vi "Configure Channel Spacing.vi"(7 "error in (no error)":errorcluster {"code" format="%.0x"}, 9 "FrequencyDifference":dbl[](array[numeric])=[20000000.0, 40000000.0, 60000000.0] format="%.2p", 10 "instrument handle":refnum<k15>) -> (0 "error out":errorcluster {"code" format="%.0x"}, 1 "FrequencyDifferenceActualSize":i32, 3 "instrument handle out":refnum<k15>)   [LabVIEW 2009, in "Keysight XSAn.lvlib"]
doc: "Sets the width of the carrier spacing. This will be the value applied to all the current slots, whether they are carriers or spaces.\n\nSupported Models: M9290A, N8973B, N8974B, N8975B, N8976B, N9000A, N9000B, N9010A, N9010B, N9020A, N9020B, N9030A, N9030B, N9038A, N9040B, N9041B, SPN9003A, SPN9026A"
uses:
  <instrlib>/Keysight XSAn/Keysight XSAn.lvlib
  AgXSAn.dll
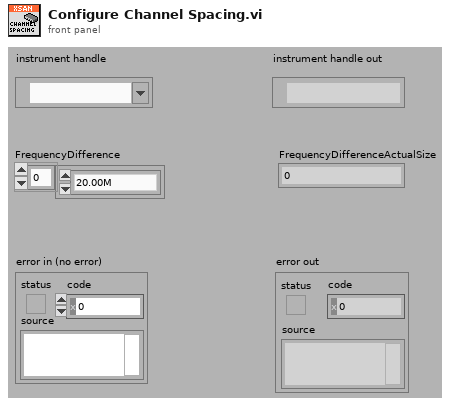
[diagram p1: front panel]
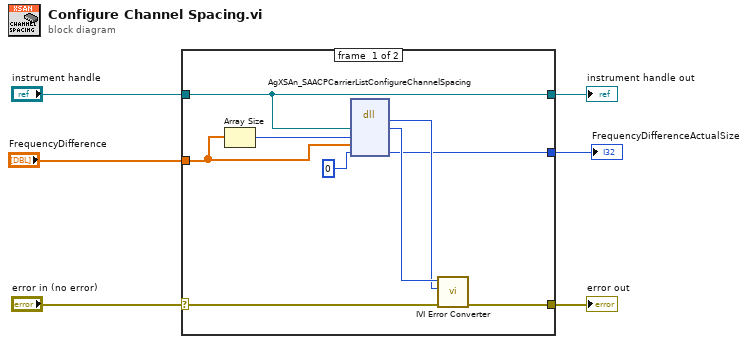
[diagram p0: block diagram]
diagram:
  n1 = case shown="No Error" "error in (no error)" {
    selector: "error in (no error)" -> [w13 w17]
    tunnel: [w12 w17] -> w6
    tunnel: "instrument handle" -> [w9 w16]
    tunnel: [w10 _] -> w3
    tunnel: [w9 w16] -> w2
    tunnel: "FrequencyDifference" -> [w8 _]
    frame #0 {
      n2 = Array Size(array=w8) -> (size(s)=w7:i32)
      n3 = dll-call lib="AgXSAn**.dll" fn="AgXSAn_SAACPCarrierListConfigureChannelSpacing"("Vi"=w9, "FrequencyDifferenceBufferSize"=w7, "FrequencyDifference"=w8, "FrequencyDifferenceActualSize"=0) -> (w14:i32, "Vi"=w15:u32, "FrequencyDifferenceActualSize"=w10:i32)  [unwired: 5 in, 2 out]
      n4 = call <instrlib>:"IVI Error Converter.vi"("error in (no error)"=w13, "IVI error code (0)"=w14, "instrument handle"=w15) -> ("error out"=w12:errorcluster)  [unwired: 7 in, 1 out]
    }
    frame #1 {
    }
  }
  "error out" <- w6
  "instrument handle out" <- w2
  "FrequencyDifferenceActualSize" <- w3
